vi "Data_get.vi"() -> ()   [LabVIEW 2009]
uses:
  <vilib>/Analysis/2dsp.llb/Real FFT.vi
  <vilib>/Analysis/NI_AALPro.lvlib
panel:
  in  "Auto":bool caption="Autosave"
  in  "FFT every#":u32=1 min=1 max=1000 step=1
  in  "#steps":u32=1 min=1 step=1
  in  "f step (MHz)":dbl=0.0003 min=0.00025 max=67.0 step=1e-06 format="%#.12f"
  in  "ps/point":T1(ring)
  in  "ns/div":T2(ring)
  out "Current sweep":u32=1 min=1 max=1000 step=1
  in  "Ext":string="ccd"
  out "f cur. (MHz)":string
  in  "Name":string="trace"
  in  "Folder":path
  in  "#Sweeps":u32=1 min=1 max=1000 step=1
  in  "Ampl. (dBm)":dbl min=-135.0 max=30.0 step=0.5 format="%#_8g"
  in  "f start (MHz)":dbl=0.0003 min=0.00025 max=67.0 step=1e-06 format="%#.12f"
  in  "Start":bool
  in  "Quit":bool
  in  "E8257D VISA Port":refnum<visa-resource-name>="GPIB0::1::INSTR"
  out "read time (ms)":u32
  out "#points":u32
  out "Busy":bool
  in  "Repetition rate (Hz)":ext=2.5
  in  "Chirp start (MHz)":ext=2.5
  in  "Filter up to (MHz)":ext=2.5
  in  "Amount of averagings":u32=10
  out "Data":dbl[](array[numeric])
  out "XY Graph 5":cluster{ext[], dbl[]}(graph)
  out "FFT (Im)":dbl[](array[numeric])
  out "FFT (Re)":dbl[](array[numeric])
  out "Final array":ext[][](array[numeric])
  out "size(s)":i32
  out "Oscilloscope Data":dbl[](array[numeric])
  in  "Channel Number":u16=1
  out "Oscilloscope graph":dbl[](graph)
  in  "Stop":bool
  in  "TDS VISA Port":refnum<visa-resource-name>="GPIB0::1::INSTR"
  # "TDS6000"
  # "E8257D"
  # "File Storage"
  # "Control"
  # "Spectrum data"
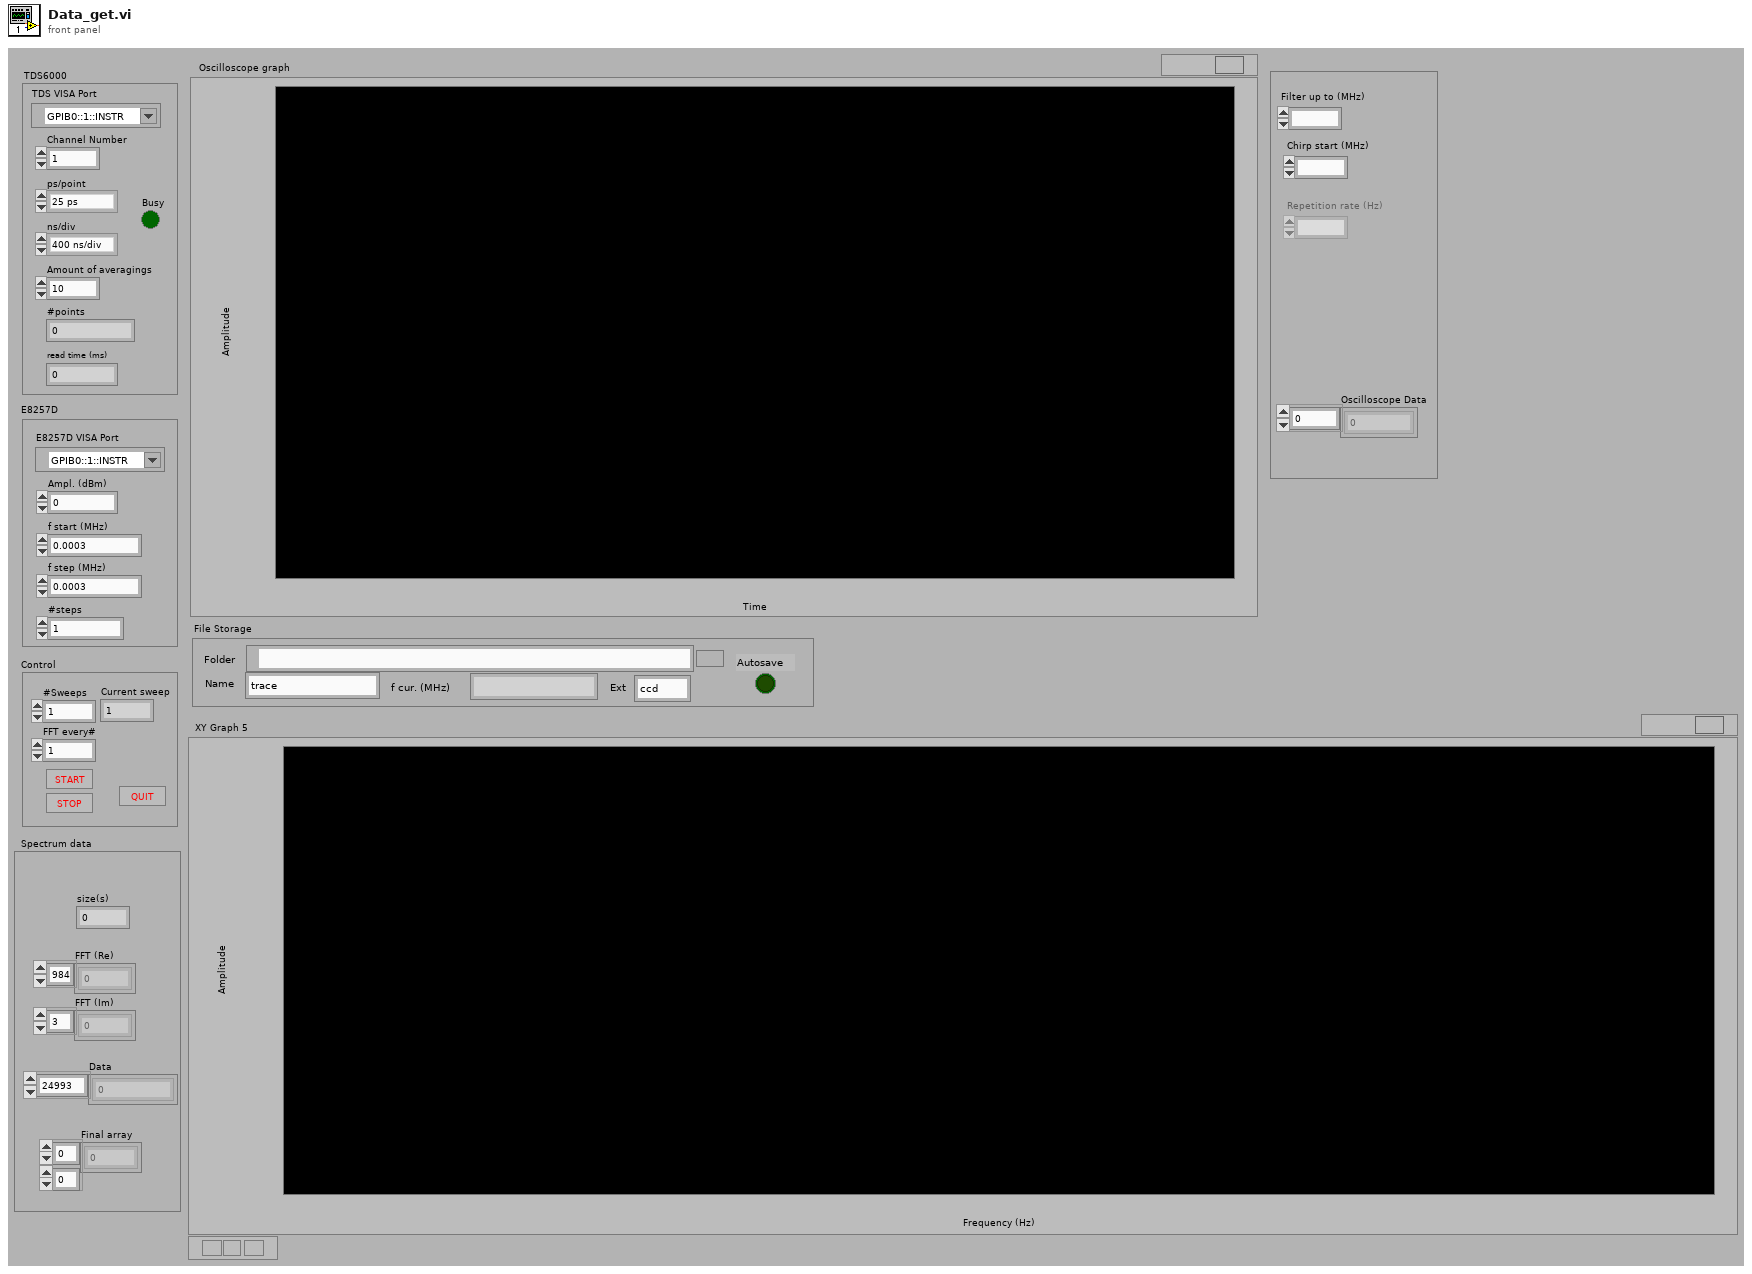
[diagram p1: front panel]
types:
  T1 = enum16{"25 ps", "50 ps", "100 ps", "200 ps", "400 ps", "800 ps", "2 ns"}
  T2 = enum16{"400 ns/div", "1 us/div", "2 us/div", "4 us/div", "10 us/div", "20 us/div"}
  T3 = enum16{"open", "replace", "create", "open or create", "replace or create", "replace or create with confirmation"}
  T4 = cluster{"Folder":path, "Name":string, "Ext":string}
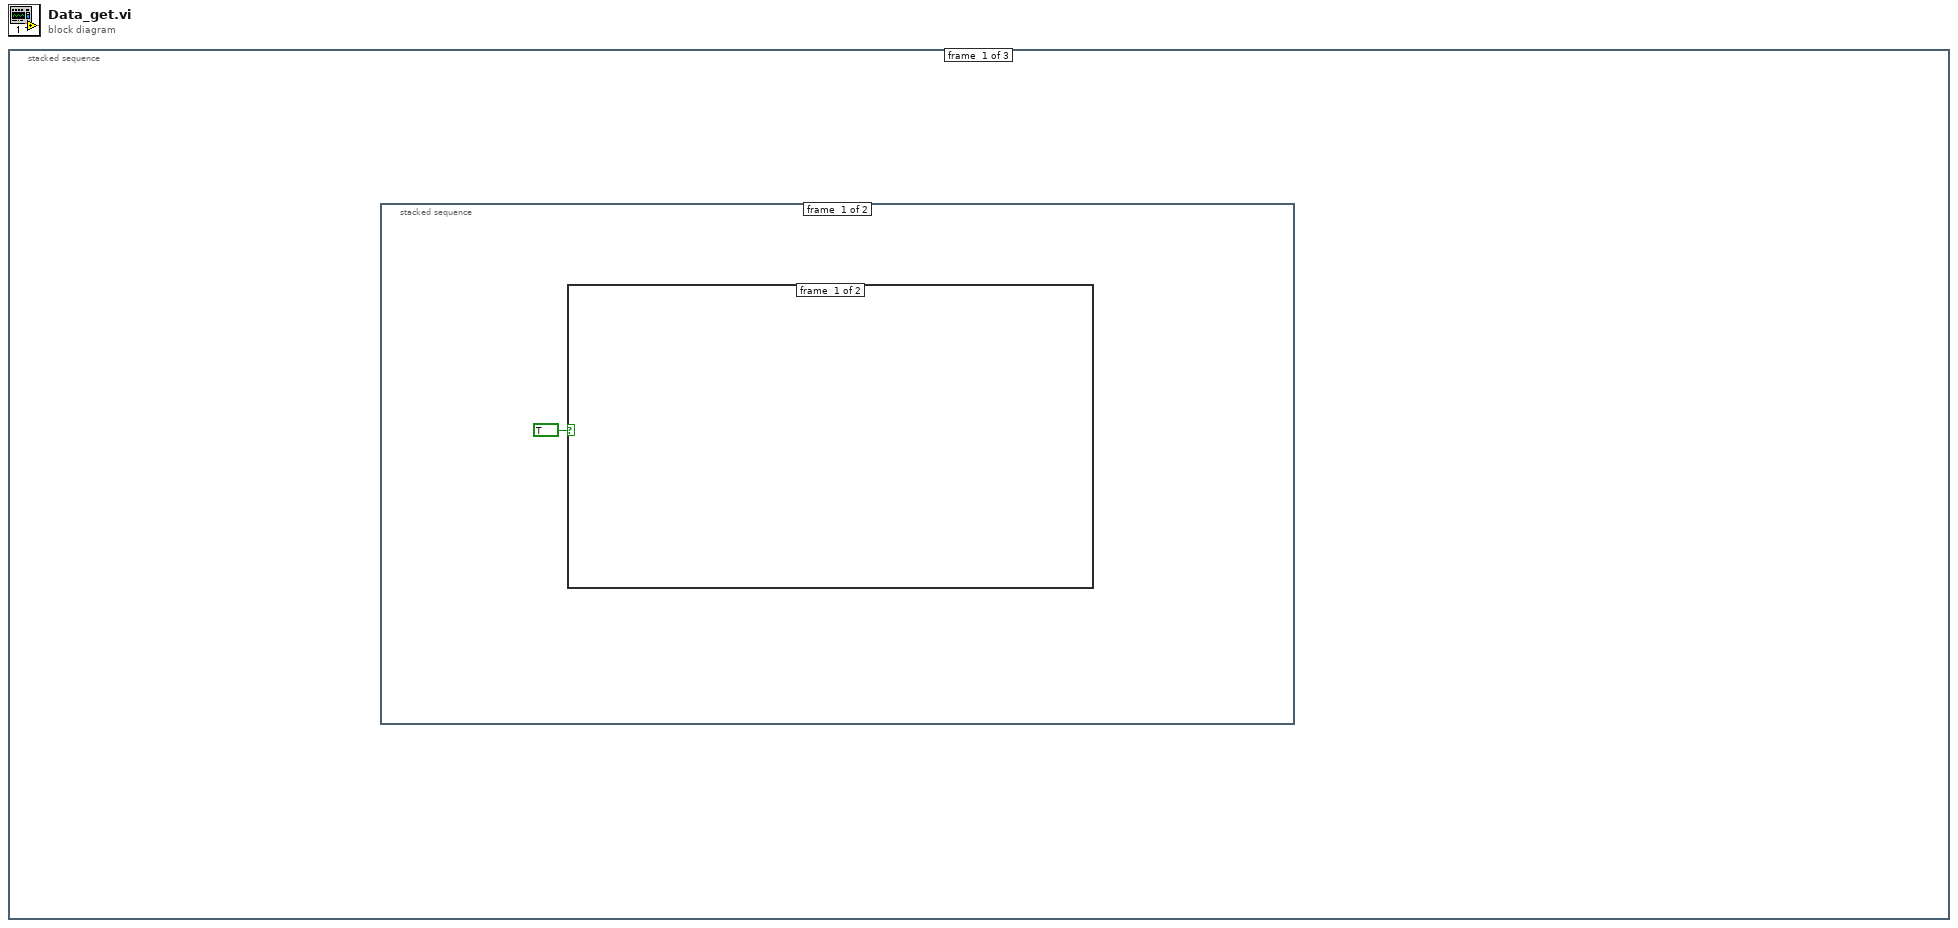
[diagram p0: block diagram]
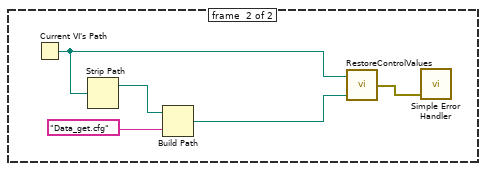
[diagram p2: hidden frame]
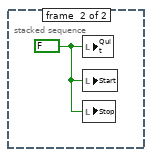
[diagram p3: hidden frame]
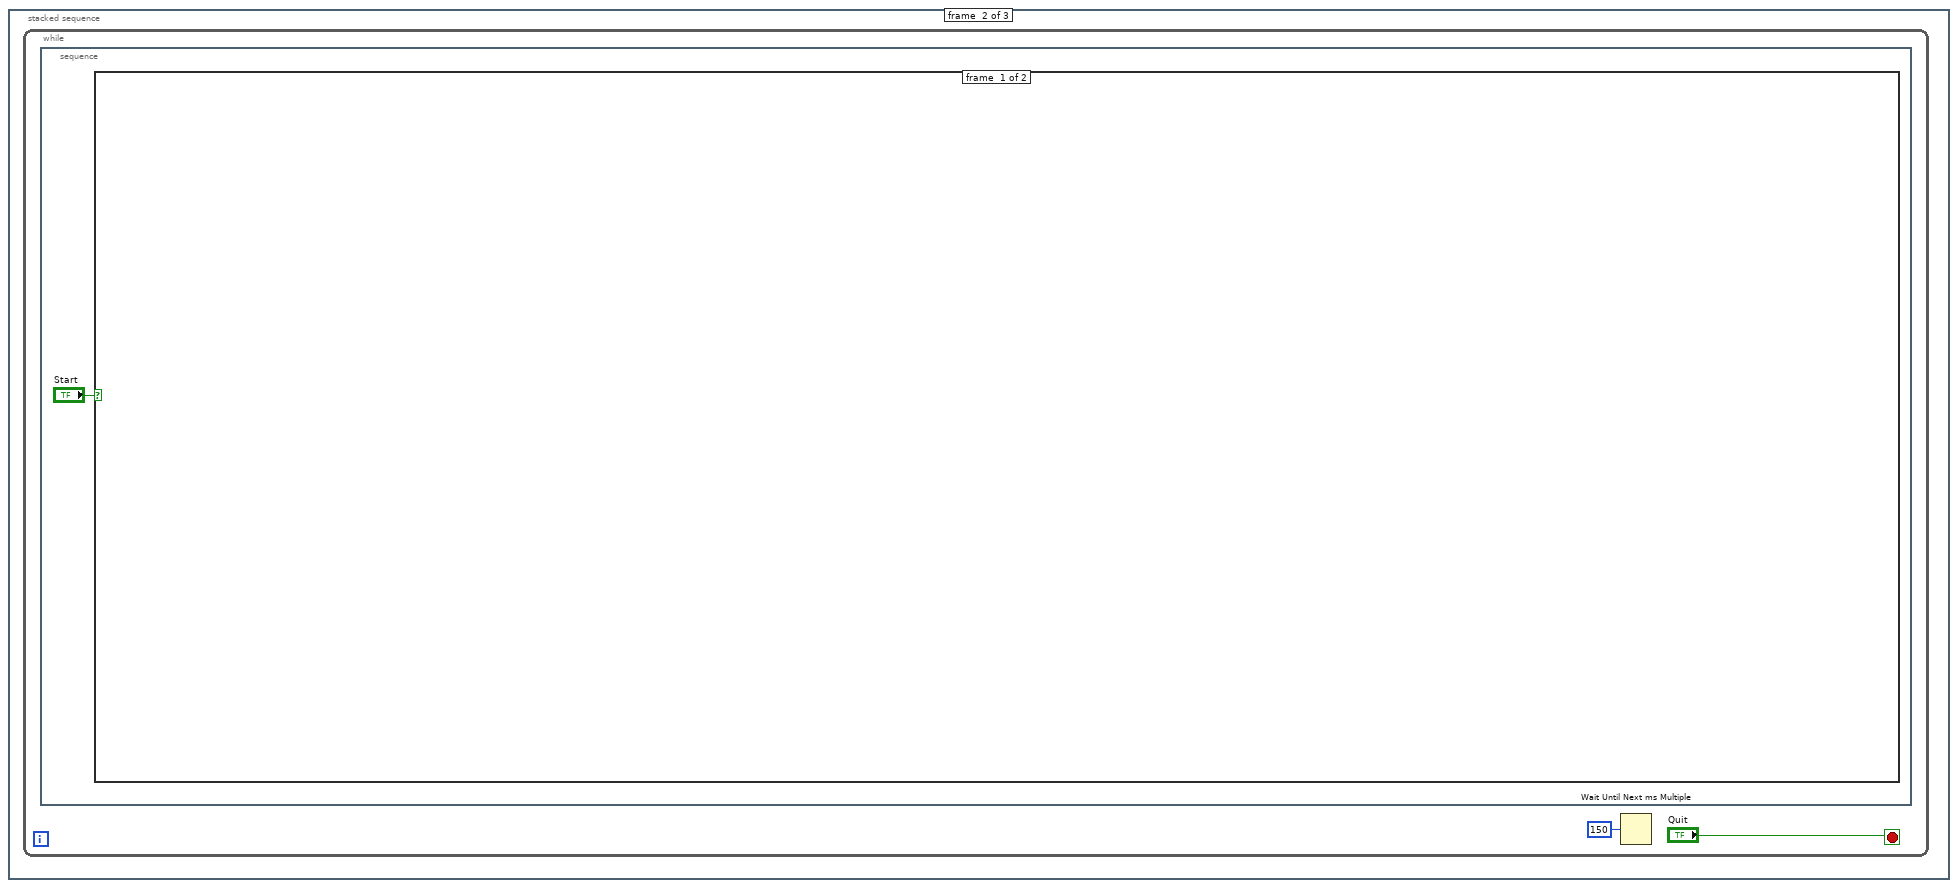
[diagram p4: hidden frame]
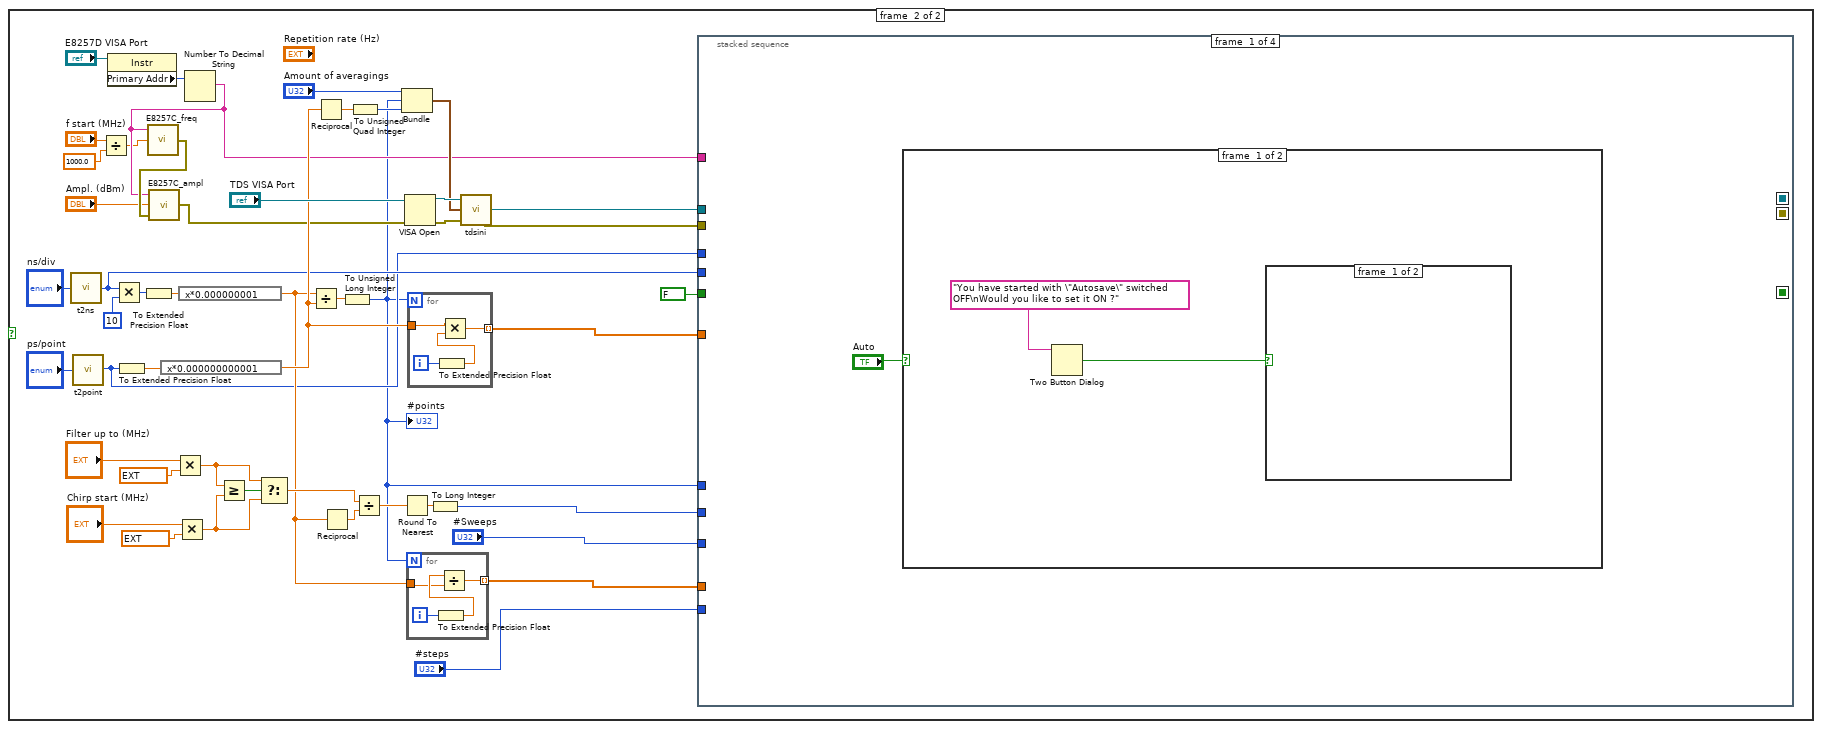
[diagram p5: hidden frame]
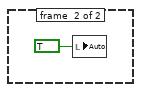
[diagram p6: hidden frame]
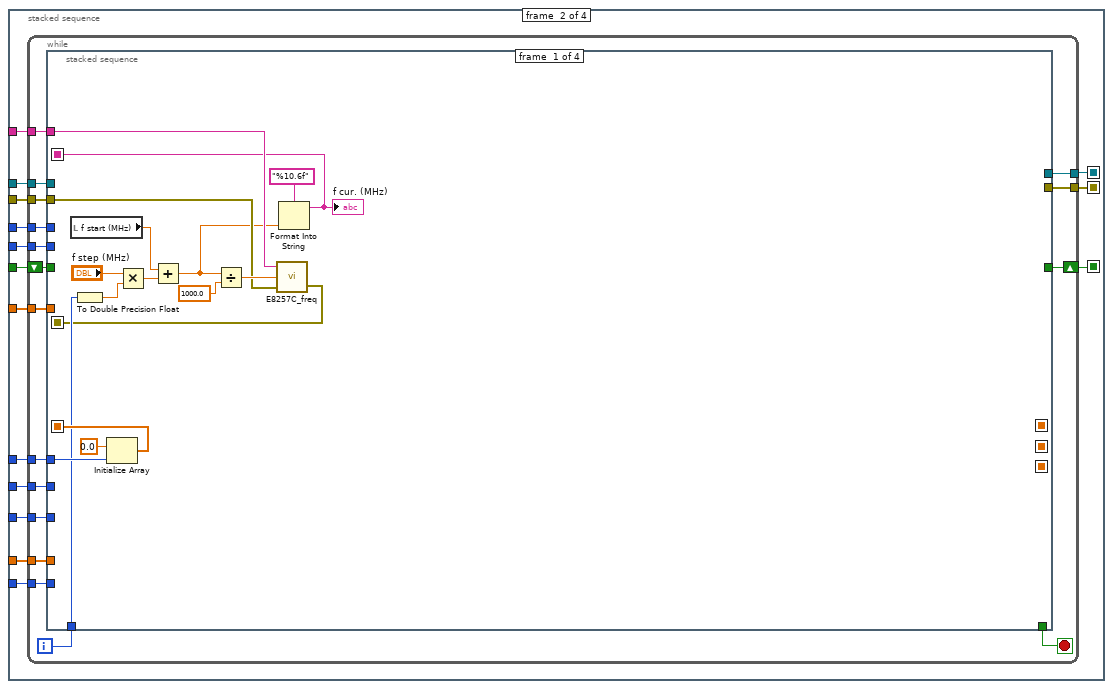
[diagram p8: hidden frame]
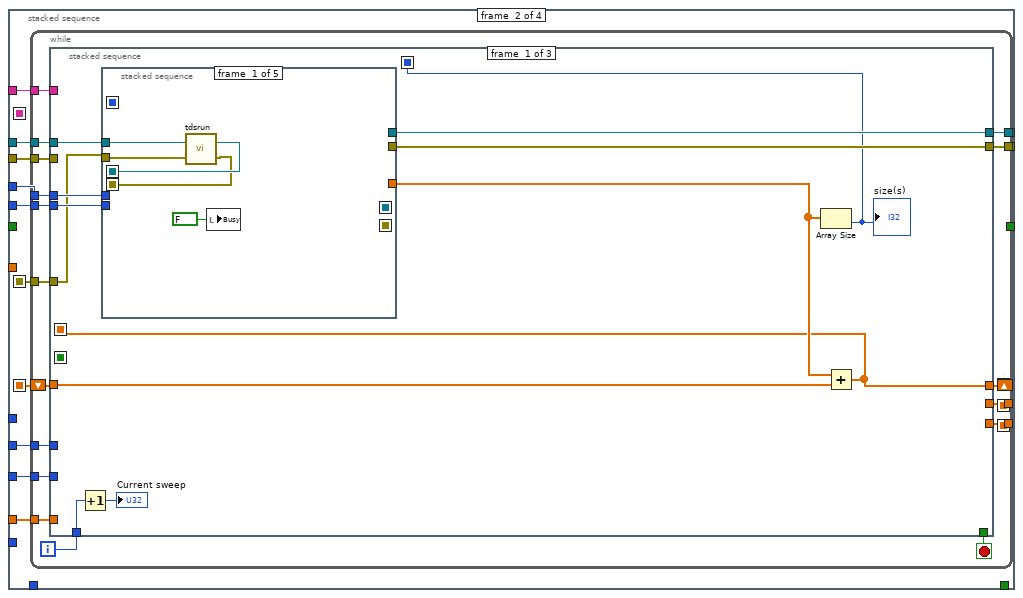
[diagram p9: hidden frame]
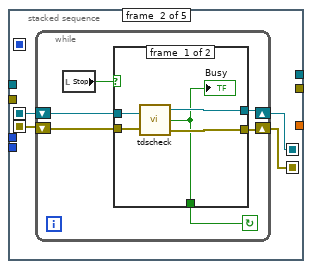
[diagram p10: hidden frame]
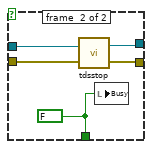
[diagram p11: hidden frame]
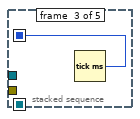
[diagram p12: hidden frame]
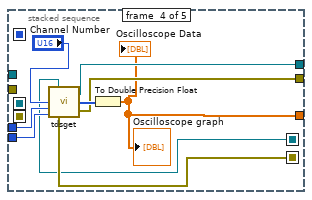
[diagram p13: hidden frame]
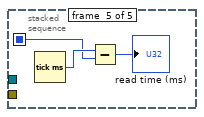
[diagram p14: hidden frame]
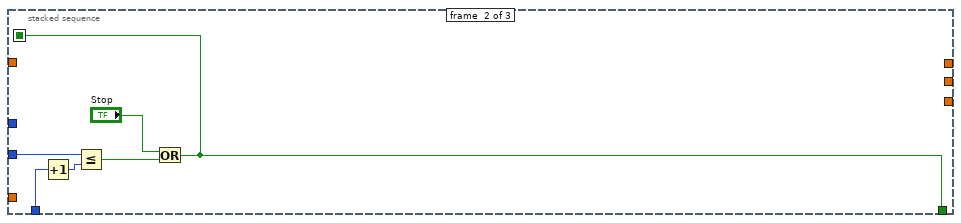
[diagram p15: hidden frame]
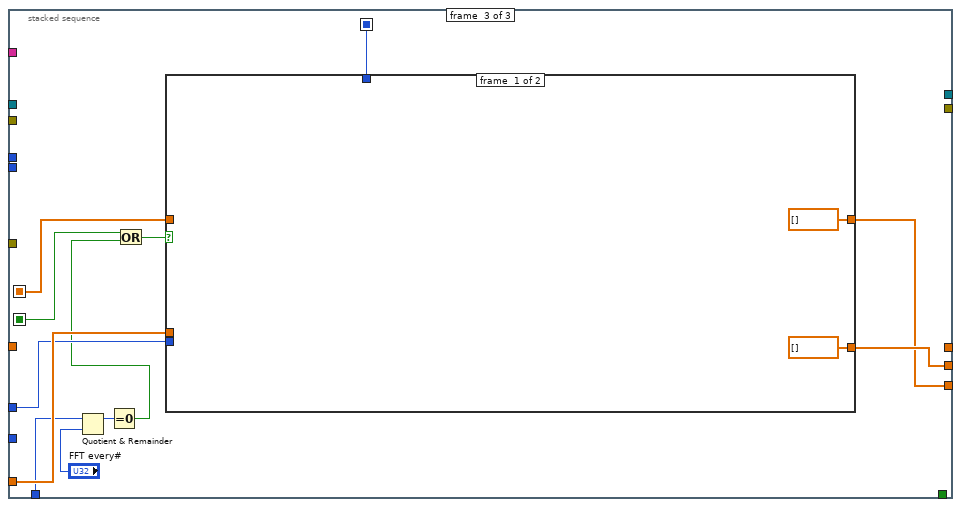
[diagram p16: hidden frame]
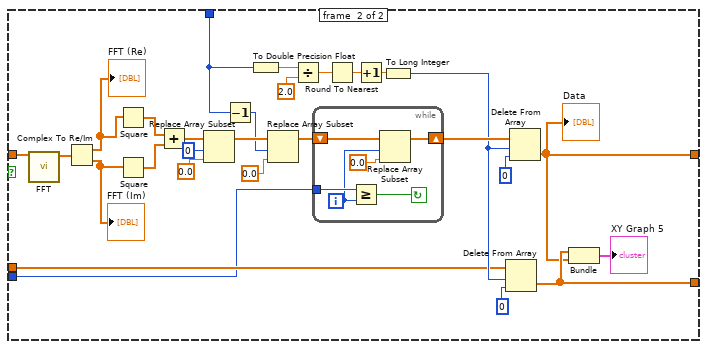
[diagram p17: hidden frame]
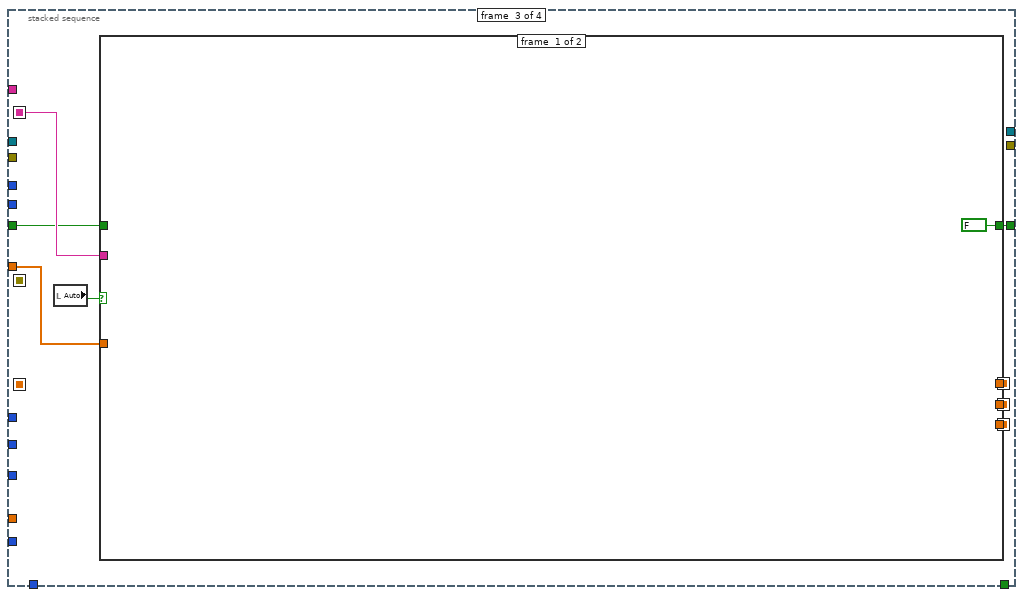
[diagram p18: hidden frame]
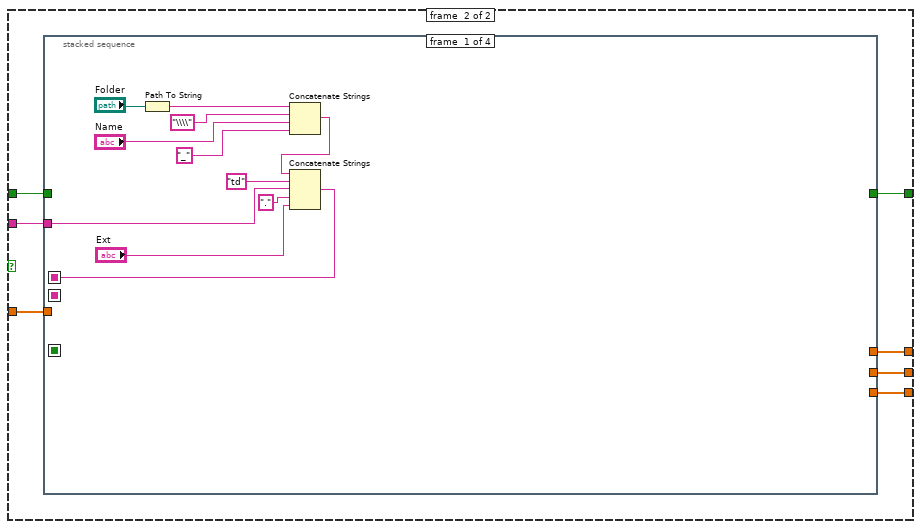
[diagram p19: hidden frame]
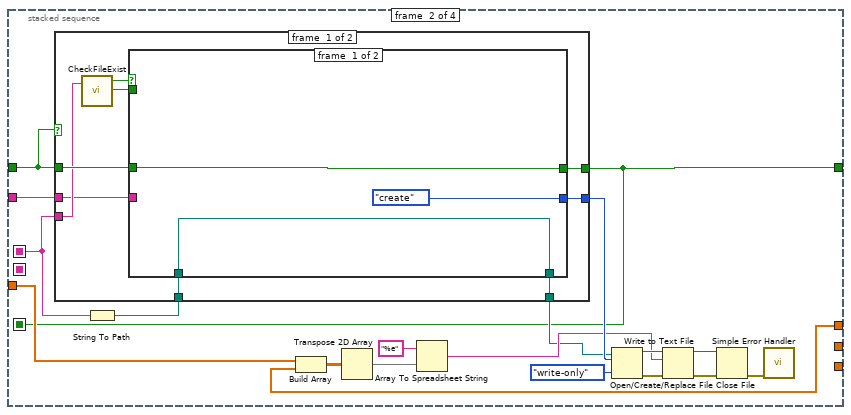
[diagram p20: hidden frame]
diagram:
  n1 = stacked-sequence {
    frame #0 {
      n2 = stacked-sequence {
        frame #0 {
          n3 = case shown="True" TRUE {
            frame #0 {
            }
            frame #1 {
              n4 = Current VI's Path() -> (path=w2:path)
              n5 = Strip Path(path=w2) -> (stripped path=w3:path)  [unwired: 1 out]
              n6 = Build Path(base path=w3, name or relative path="Data_get.cfg") -> (appended path=w5:path)
              n7 = call "RestoreControlValues.vi"("file path"=w5, "vi path"=w2) -> ("error out"=w4:errorcluster)
              n8 = call <vilib>:"Simple Error Handler.vi"("error in (no error)"=w4) -> ()  [unwired: 4 in, 5 out]
            }
          }
        }
        frame #1 {
          w7 = FALSE ("Quit")
          n9 = local write "Quit"(w7) -> ()
          n10 = local write "Start"(w7) -> ()
          n11 = local write "Stop"(w7) -> ()
        }
      }
    }
    frame #1 {
      n12 = while {
        stop <- "Quit" stop-if-true
        n13 = stacked-sequence {
          frame #0 {
            n14 = case shown="True" "Start" {
              frame #0 {
              }
              frame #1 {
                n15 = call "t2ns.vi"("t/div"="ns/div") -> ("ns/div"=w17:u32)
                n16 = call "t2point.vi"("t/point"="ps/point") -> ("ps/point"=w15:u32)
                n17 = Divide(x="f start (MHz)", y=1000.0) -> (x/y=w20:dbl)
                n18 = property class="Instr"(reference="E8257D VISA Port") -> ("Primary Addr"=w27:u16)  [unwired: 1 in, 2 out]
                n19 = Multiply(x=w17, y=u32 10) -> (x*y=w51:u32)
                n20 = To Extended Precision Float(1:w15) -> (0:w48:ext)
                n21 = To Extended Precision Float(1:w51) -> (0:w49:ext)
                n22 = expression code="x*0.000000000001"(w48) -> (w33:ext)
                n23 = Multiply(x="Filter up to (MHz)", y=ext 1000000.0) -> (x*y=w39:ext)
                n24 = Multiply(x="Chirp start (MHz)", y=ext 1000000.0) -> (x*y=w36:ext)
                n25 = expression code="x*0.000000001"(w49) -> (w29:ext)
                n26 = Number To Decimal String(number=w27) -> (decimal integer string=w24:string)  [unwired: 1 in]
                n27 = call "E8257C_freq.vi"("Frequency GHz"=w20, "GPIB address"=w24) -> ("error out"=w25:errorcluster)  [unwired: 1 in]
                n28 = call "E8257C_ampl.vi"("error in"=w25, "Amplitude dBm"="Ampl. (dBm)", "GPIB address"=w24) -> ("error out"=w23:errorcluster)
                n29 = Greater Or Equal?(x=w39, y=w36) -> (x >= y?=w47:bool)
                n30 = Select(t=w39, s=w47, f=w36) -> (s? t:f=w45:ext)
                n31 = Divide(x=w29, y=w33) -> (x/y=w50:ext)
                n32 = Reciprocal(x=w33) -> (1/x=w31:ext)
                n33 = Reciprocal(x=w29) -> (1/x=w46:ext)
                n34 = To Unsigned Long Integer(number=w50) -> (unsigned 32bit integer=w13:u32)
                "#points" <- w13
                n35 = To Unsigned Quad Integer(1:w31) -> (0:w32:u64)
                n36 = Divide(x=w45, y=w46) -> (x/y=w44:ext)
                n37 = Bundle("Amount of averagings"="Amount of averagings", w13, w32) -> (w34:cluster{"Amount of averagings ":u32, u32, u64})  [unwired: 1 in]
                n38 = Round To Nearest(number=w44) -> (nearest integer value=w43:ext)
                n39 = VISA Open(error in (no error)=w23, VISA resource name="TDS VISA Port") -> (VISA resource name=w54:refnum<visa-resource-name>, error out=w55:errorcluster)  [unwired: 3 in]
                n40 = for {
                  N: w13 -> [_]
                  tunnel: w29 -> [w420]
                  tunnel: [w422] -> w30 mode=indexing
                  i -> [w423]
                  n41 = To Extended Precision Float(1:w423) -> (0:w421:ext)
                  n42 = Divide(x=w421, y=w420) -> (x/y=w422:ext)
                }
                n43 = for {
                  N: w13 -> [_]
                  tunnel: w33 -> [w425]
                  tunnel: [w424] -> w18 mode=indexing
                  i -> [w427]
                  n44 = To Extended Precision Float(1:w427) -> (0:w426:ext)
                  n45 = Multiply(x=w425, y=w426) -> (x*y=w424:ext)
                }
                n46 = To Long Integer(number=w43) -> (32bit integer=w42:i32)
                n47 = call "tdsini.vi"("Error In (No Error)"=w55, "Acq_par"=w34, "VISA Port In"=w54) -> ("Error Out"=w56:errorcluster, "VISA Port Out"=w57:refnum<visa-resource-name>)
                n48 = stacked-sequence {
                  seq-local: [_ w68 _ _] -> [_ _ w381 _]
                  seq-local: [_ w67 _ _] -> [_ _ w380 _]
                  seq-local: [_ w62 _ _] -> [_ _ _ w382]
                  tunnel: w57 -> [_ w76 _ _]
                  tunnel: w56 -> [_ w75 _ _]
                  tunnel: w15 -> [_ w74 _ _]
                  tunnel: w17 -> [_ w73 _ _]
                  tunnel: w42 -> [_ w72 _ _]
                  tunnel: w30 -> [_ w71 _ _]
                  tunnel: w24 -> [_ w70 w378 _]
                  tunnel: "#Sweeps" -> [_ w69 _ _]
                  tunnel: w18 -> [_ w64 _ _]
                  tunnel: w13 -> [_ w66 _ _]
                  tunnel: "#steps" -> [_ w65 _ _]
                  tunnel: FALSE -> [_ w63 _ _]
                  frame #0 {
                    n49 = case shown="False" "Auto" {
                      frame #0 {
                        n50 = Two Button Dialog(message="You have started with \"Autosave\" switched OFF\nWould you like to set it ON ?") -> (T button?=w59:bool)  [unwired: 2 in]
                        n51 = case shown="True" w59 {
                          frame #0 {
                          }
                          frame #1 {
                            n52 = local write "Auto"(TRUE) -> ()
                          }
                        }
                      }
                      frame #1 {
                      }
                    }
                  }
                  frame #1 {
                    n53 = while {
                      tunnel: w76 -> [w93]
                      tunnel: w75 -> [w92]
                      tunnel: w74 -> [w91]
                      tunnel: w73 -> [w90]
                      tunnel: w72 -> [w89]
                      tunnel: w71 -> [w88]
                      tunnel: w70 -> [w87]
                      tunnel: w69 -> [w86]
                      tunnel: [w85] -> w68
                      tunnel: [w84] -> w67
                      tunnel: w66 -> [w83]
                      tunnel: w65 -> [w81]
                      tunnel: w64 -> [w79]
                      shift-right: [w77] -> w62
                      shift-left: w63 -> [w78]
                      i -> [w82]
                      stop <- w80 stop-if-true
                      n54 = stacked-sequence {
                        seq-local: [w108 _ _ _] -> [_ w114 _ _]
                        seq-local: [w97 _ _ _] -> [_ w113 _ _]
                        seq-local: [_ w112 _ _] -> [_ _ w252 _]
                        seq-local: [_ w111 _ _] -> [_ _ w251 _]
                        seq-local: [_ w110 _ _] -> [_ _ w250 _]
                        seq-local: [w94 _ _ _] -> [_ _ w249 _]
                        tunnel: w93 -> [_ w124 _ _]
                        tunnel: w92 -> [w98 w123 _ _]
                        tunnel: w91 -> [_ w122 _ _]
                        tunnel: w90 -> [_ w121 _ _]
                        tunnel: w89 -> [_ w120 _ _]
                        tunnel: w88 -> [_ w119 _ _]
                        tunnel: w87 -> [w99 w118 _ _]
                        tunnel: w86 -> [_ w117 _ _]
                        tunnel: [_ w116 _ _] -> w85
                        tunnel: [_ w115 _ _] -> w84
                        tunnel: w83 -> [w107 _ _ _]
                        tunnel: w82 -> [w102 _ _ w374]
                        tunnel: w81 -> [_ _ _ w373]
                        tunnel: [_ _ _ w372] -> w80
                        tunnel: w79 -> [_ _ w253 _]
                        tunnel: w78 -> [_ _ w247 _]
                        tunnel: [_ _ w246 _] -> w77
                        frame #0 {
                          n55 = local read "f start (MHz)"() -> (w100:dbl)
                          n56 = To Double Precision Float(number=w102) -> (double precision float=w103:dbl)
                          n57 = Initialize Array(0.0 ("element"), w107) -> (w108:dbl[])
                          n58 = Multiply(x="f step (MHz)", y=w103) -> (x*y=w101:dbl)
                          n59 = Add(x=w100, y=w101) -> (x+y=w96:dbl)
                          n60 = Divide(x=w96, y=1000.0) -> (x/y=w106:dbl)
                          n61 = call "E8257C_freq.vi"("error in"=w98, "Frequency GHz"=w106, "GPIB address"=w99) -> ("error out"=w97:errorcluster)
                          n62 = Format Into String(format string="%10.6f", w96) -> (resulting string=w94:string)  [unwired: 2 in, 1 out]
                          "f cur. (MHz)" <- w94
                        }
                        frame #1 {
                          n63 = while {
                            tunnel: [w138] -> w115
                            tunnel: [w139] -> w116
                            tunnel: w123 -> [w140]
                            tunnel: w124 -> [w141]
                            tunnel: w122 -> [w137]
                            tunnel: w121 -> [w136]
                            tunnel: w119 -> [w134]
                            tunnel: w120 -> [w135]
                            tunnel: w118 -> [w131]
                            tunnel: w117 -> [w130]
                            shift-right: [w128] -> w112
                            shift-left: w114 -> [w129]
                            tunnel: [w127] -> w111
                            tunnel: w113 -> [w126]
                            tunnel: [w125] -> w110
                            i -> [w133]
                            stop <- w132 stop-if-true
                            n64 = stacked-sequence {
                              seq-local: [w142 _ _] -> [_ _ w209]
                              seq-local: [w143 _ _] -> [_ _ w208]
                              seq-local: [_ w192 _] -> [_ _ w199]
                              tunnel: w141 -> [w153 _ _]
                              tunnel: w140 -> [_ _ _]
                              tunnel: [w152 _ _] -> w139
                              tunnel: [w151 _ _] -> w138
                              tunnel: w137 -> [w150 _ _]
                              tunnel: w136 -> [w149 _ _]
                              tunnel: w135 -> [_ _ w206]
                              tunnel: w134 -> [_ _ w207]
                              tunnel: w133 -> [w146 w197 w203]
                              tunnel: [_ w192 _] -> w132
                              tunnel: w131 -> [_ _ _]
                              tunnel: w130 -> [_ w194 _]
                              tunnel: w129 -> [w148 _ _]
                              tunnel: [w143 _ _] -> w128
                              tunnel: [_ _ w205] -> w127
                              tunnel: w126 -> [w145 _ _]
                              tunnel: [_ _ w204] -> w125
                              frame #0 {
                                n65 = Increment(x=w146) -> (x+1=→"Current sweep":i32)
                                n66 = stacked-sequence {
                                seq-local: [w156 _ _ _ _] -> [_ w162 _ _ _]
                                seq-local: [w155 _ _ _ _] -> [_ w161 _ _ _]
                                seq-local: [_ w159 _ _ _] -> [_ _ _ w181 _]
                                seq-local: [_ w160 _ _ _] -> [_ _ _ w180 _]
                                seq-local: [_ _ w179 _ _] -> [_ _ _ _ w190]
                                tunnel: w153 -> [w157 _ _ _ _]
                                tunnel: w145 -> [w158 _ _ _ _]
                                tunnel: [_ _ _ w187 _] -> w152
                                tunnel: [_ _ _ w186 _] -> w151
                                tunnel: w150 -> [_ _ _ w184 _]
                                tunnel: w149 -> [_ _ _ w183 _]
                                tunnel: [_ _ _ w182 _] -> w144
                                frame #0 {
                                n67 = call "tdsrun.vi"("Error In (No Error)"=w158, "VISA Port In"=w157) -> ("Error Out"=w155:errorcluster, "VISA Port Out"=w156:refnum<visa-resource-name>)
                                n68 = local write "Busy"(FALSE ("Busy")) -> ()
                                }
                                frame #1 {
                                n69 = while {
                                shift-right: [w166] -> w160
                                shift-left: w162 -> [w167]
                                shift-right: [w165] -> w159
                                shift-left: w161 -> [w168]
                                stop <- w164 continue-if-true
                                n70 = local read "Stop"() -> (w163:bool)
                                n71 = case shown="True" w163 {
                                tunnel: w168 -> [w173 w177]
                                tunnel: w167 -> [w172 w178]
                                tunnel: [w171 w175] -> w166
                                tunnel: [w170 w176] -> w165
                                tunnel: [w169 w174] -> w164
                                frame #0 {
                                n72 = call "tdscheck.vi"("VISA Port In"=w172, "Error In (No Error)"=w173) -> ("VISA Port Out"=w171:refnum<visa-resource-name>, "busy"=w169:bool, "Error Out"=w170:errorcluster)
                                "Busy" <- w169
                                }
                                frame #1 {
                                w174 = FALSE ("busy")
                                n73 = call "tdsstop.vi"("Error In (No Error)"=w177, "VISA Port In"=w178) -> ("Error Out"=w176:errorcluster, "VISA Port Out"=w175:refnum<visa-resource-name>)
                                n74 = local write "Busy"(w174) -> ()
                                }
                                }
                                }
                                }
                                frame #2 {
                                n75 = Tick Count (ms)() -> (millisecond timer value=w179:u32)
                                }
                                frame #3 {
                                n76 = call "tdsget.vi"("VISA Port In"=w180, "Channel Number"="Channel Number", "ps/point"=w184, "ns/div"=w183, "Error In (No Error)"=w181) -> ("VISA Port Out"=w187:refnum<visa-resource-name>, "TDS Data"=w188:u16[], "Error Out"=w186:errorcluster)  [unwired: 8 in]
                                n77 = To Double Precision Float(number=w188) -> (double precision float=w182:dbl[])
                                "Oscilloscope graph" <- w182
                                "Oscilloscope Data" <- w182
                                }
                                frame #4 {
                                n78 = Tick Count (ms)() -> (millisecond timer value=w191:u32)
                                n79 = Subtract(x=w191, y=w190) -> (x-y=→"read time (ms)":u32)
                                }
                                }
                                n80 = Array Size(array=w144) -> (size(s)=w142:i32)
                                "size(s)" <- w142
                                n81 = Add(x=w144, y=w148) -> (x+y=w143:dbl[])
                              }
                              frame #1 {
                                n82 = Increment(x=w197) -> (x+1=w193:i32)
                                n83 = Less Or Equal?(x=w194, y=w193) -> (x <= y?=w196:bool)
                                n84 = Or(x="Stop", y=w196) -> (x .or. y?=w192:bool)
                              }
                              frame #2 {
                                n85 = Quotient & Remainder(x=w203, y="FFT every#") -> (x-y*floor(x/y)=w201:u32)  [unwired: 1 out]
                                n86 = Equal To 0?(x=w201) -> (x = 0?=w198:bool)
                                n87 = Or(x=w199, y=w198) -> (x .or. y?=w200:bool)
                                n88 = case shown="True" w200 {
                                tunnel: w209 -> [_ w217]
                                tunnel: w208 -> [_ w216]
                                tunnel: w207 -> [_ w215]
                                tunnel: w206 -> [_ w214]
                                tunnel: [ext[] [] w213] -> w205
                                tunnel: [dbl[] [] w212] -> w204
                                frame #0 {
                                }
                                frame #1 {
                                n89 = call-poly <vilib>:"FFT.vi"("X"=w216) -> ("FFT {X}"=w239:cdb[])  [unwired: 9 in, 1 out]
                                n90 = Complex To Re/Im(x + iy=w239) -> (x=w238:dbl[], y=w237:dbl[])
                                "FFT (Re)" <- w238
                                "FFT (Im)" <- w237
                                n91 = Square(x=w238) -> (x^2=w236:dbl[])
                                n92 = Square(x=w237) -> (x^2=w235:dbl[])
                                n93 = Add(x=w236, y=w235) -> (x+y=w231:dbl[])
                                n94 = Replace Array Subset(array=w231, new element=0.0 ("new element/subarray"), index=0) -> (w230:dbl[])
                                n95 = Decrement(x=w217) -> (x-1=w229:i32)
                                n96 = To Double Precision Float(number=w217) -> (double precision float=w225:dbl)
                                n97 = Replace Array Subset(array=w230, new element=0.0 ("new element/subarray"), index=w229) -> (w227:dbl[])
                                n98 = Divide(x=w225, y=2.0) -> (x/y=w223:dbl)
                                n99 = while {
                                tunnel: w214 -> [w244]
                                shift-right: [w242] -> w226
                                shift-left: w227 -> [w243]
                                i -> [w241]
                                stop <- w245 continue-if-true
                                n100 = Greater Or Equal?(x=w244, y=w241) -> (x >= y?=w245:bool)
                                n101 = Replace Array Subset(array=w243, new element=0.0 ("new element/subarray"), index=w241) -> (w242:dbl[])
                                }
                                n102 = Round To Nearest(number=w223) -> (nearest integer value=w222:dbl)
                                n103 = Increment(x=w222) -> (x+1=w221:dbl)
                                n104 = To Long Integer(number=w221) -> (32bit integer=w218:i32)
                                n105 = Delete From Array(array=w215, length=w218, index=0) -> (deleted portion=w213:ext[])  [unwired: 1 out]
                                n106 = Delete From Array(array=w226, length=w218, index=0) -> (deleted portion=w212:dbl[])  [unwired: 1 out]
                                "Data" <- w212
                                n107 = Bundle(w213, w212) -> (→"XY Graph 5":cluster{ext[], dbl[]})  [unwired: 1 in]
                                }
                                }
                              }
                            }
                          }
                        }
                        frame #2 {
                          n108 = local read "Auto"() -> (w248:bool)
                          n109 = case shown="True" w248 {
                            tunnel: w253 -> [_ w261]
                            tunnel: w252 -> [_ w260]
                            tunnel: w251 -> [_ w259]
                            tunnel: w250 -> [_ w258]
                            tunnel: w249 -> [_ w257]
                            tunnel: w247 -> [_ w256]
                            tunnel: [FALSE w255] -> w246
                            frame #0 {
                            }
                            frame #1 {
                              n110 = stacked-sequence {
                                seq-local: [w262 _ _ _] -> [_ w287 _ _]
                                seq-local: [_ _ w342 _] -> [_ _ _ w363]
                                seq-local: [_ w274 _ _] -> [_ _ _ w354]
                                tunnel: w261 -> [_ w289 _ _]
                                tunnel: w260 -> [_ w276 _ _]
                                tunnel: w259 -> [_ _ _ w366]
                                tunnel: w258 -> [_ _ _ w365]
                                tunnel: w257 -> [w264 w275 w344 _]
                                tunnel: w256 -> [_ w279 _ _]
                                tunnel: [_ w274 _ _] -> w255
                                frame #0 {
                                n111 = Path To String(path="Folder") -> (string=w272:string)
                                n112 = Concatenate Strings(w272, "\\\\" ("string"), "Name", "_") -> (w263:string)
                                n113 = Concatenate Strings(w263, "td", w264, ".", "Ext") -> (w262:string)
                                }
                                frame #1 {
                                n114 = String To Path(string=w287) -> (path=w278:path)
                                n115 = case shown="False" w279 {
                                tunnel: w287 -> [w293 _]
                                tunnel: [w298 w340] -> w274
                                tunnel: [w296 T3."replace or create" ("operation (0:open)")] -> w281
                                tunnel: w279 -> [w297 w340]
                                tunnel: w278 -> [w295 w339]
                                tunnel: [w294 w339] -> w277
                                tunnel: w275 -> [w292 _]
                                frame #0 {
                                n116 = call "CheckFileExist.vi"("Path"=w293) -> ("Exist"=w300:bool, "Overwrite"=w299:bool)  [unwired: 1 in, 1 out]
                                n117 = case shown="True" w300 {
                                tunnel: w299 -> [_ w309]
                                tunnel: [w303 w307] -> w298
                                tunnel: w297 -> [w303 _]
                                tunnel: [T3."create" ("operation (0:open)") w308] -> w296
                                tunnel: w295 -> [w301 w306]
                                tunnel: [w301 w305] -> w294
                                tunnel: w292 -> [_ w304]
                                frame #0 {
                                }
                                frame #1 {
                                n118 = case shown="True" w309 {
                                tunnel: [w312 T3."replace or create" ("operation (0:open)")] -> w308
                                tunnel: [w313 TRUE] -> w307
                                tunnel: w306 -> [_ w336]
                                tunnel: [w310 w336] -> w305
                                tunnel: w304 -> [w311 _]
                                frame #0 {
                                n119 = stacked-sequence {
                                tunnel: [_ _ FALSE] -> w313
                                tunnel: [_ _ T3."create" ("operation (0:open)")] -> w312
                                tunnel: w311 -> [_ w325 _]
                                tunnel: [_ w322 _] -> w310
                                frame #0 {
                                n120 = local read "Folder"() -> (w321:path)
                                n121 = local read "Name"() -> (w320:string)
                                n122 = local read "Ext"() -> (w319:string)
                                n123 = Bundle("Folder"=w321, "Name"=w320, "Ext"=w319) -> (w318:T4)  [unwired: 1 in]
                                n124 = call "ChangeFileName.vi"("input par"=w318) -> ("output par"=w317:T4)  [unwired: 1 out]
                                n125 = Unbundle(w317) -> ("Folder"=w316:path, "Name"=w315:string, "Ext"=w314:string)
                                n126 = local write "Folder"(w316) -> ()
                                n127 = local write "Name"(w315) -> ()
                                n128 = local write "Ext"(w314) -> ()
                                }
                                frame #1 {
                                n129 = local read "Folder"() -> (w330:path)
                                n130 = local read "Name"() -> (w329:string)
                                n131 = local read "Ext"() -> (w324:string)
                                n132 = Path To String(path=w330) -> (string=w333:string)
                                n133 = Concatenate Strings(w333, "\\\\" ("string"), w329, "_") -> (w326:string)
                                n134 = Concatenate Strings(w326, "td", w325, ".", w324) -> (w323:string)
                                n135 = String To Path(string=w323) -> (path=w322:path)
                                }
                                frame #2 {
                                }
                                }
                                }
                                frame #1 {
                                }
                                }
                                }
                                }
                                }
                                frame #1 {
                                }
                                }
                                n136 = Build Array(w289, w276) -> (w291:ext[][])
                                n137 = Transpose 2D Array(2D array=w291) -> (transposed array=w288:ext[][])
                                n138 = Array To Spreadsheet String(array=w288, 3:"%e") -> (spreadsheet string=w280:string)  [unwired: 1 in]
                                n139 = Open/Create/Replace File(file path (use dialog)=w277, operation (0:open)=w281, access (0:read/write)=enum16{"read/write", "read-only", "write-only"}."write-only") -> (refnum out=w283:refnum<file>, error out=w286:errorcluster)  [unwired: 3 in, 1 out]
                                n140 = Write to Text File(file (use dialog)=w283, text=w280, error in=w286) -> (refnum out=w284:refnum<file>, error out=w285:errorcluster)  [unwired: 1 in, 1 out]
                                n141 = Close File(refnum=w284, error in=w285) -> (error out=w273:errorcluster)  [unwired: 1 out]
                                n142 = call <vilib>:"Simple Error Handler.vi"("error in (no error)"=w273) -> ()  [unwired: 4 in, 5 out]
                                }
                                frame #2 {
                                n143 = local read "Folder"() -> (w346:path)
                                n144 = local read "Name"() -> (w345:string)
                                n145 = local read "Ext"() -> (w343:string)
                                n146 = Path To String(path=w346) -> (string=w352:string)
                                n147 = Concatenate Strings(w352, "\\\\" ("string"), w345, "_") -> (w347:string)
                                n148 = Concatenate Strings(w347, "sd", w344, ".", w343) -> (w342:string)
                                }
                                frame #3 {
                                n149 = To Extended Precision Float(1:w365) -> (0:w367:ext[])
                                n150 = String To Path(string=w363) -> (path=w356:path)
                                n151 = case shown="True" w354 {
                                tunnel: [T3."replace or create with confirmation" ("operation (0:open)") T3."replace or create" ("operation (0:open)")] -> w355
                                frame #0 {
                                }
                                frame #1 {
                                }
                                }
                                n152 = Build Array(w366, w367) -> (w364:ext[][])
                                n153 = Transpose 2D Array(2D array=w364) -> (transposed array=w368:ext[][])
                                "Final array" <- w368
                                n154 = Array To Spreadsheet String(array=w368, 3:"%e") -> (spreadsheet string=w357:string)  [unwired: 1 in]
                                n155 = Open/Create/Replace File(file path (use dialog)=w356, operation (0:open)=w355, access (0:read/write)=enum16{"read/write", "read-only", "write-only"}."write-only") -> (refnum out=w359:refnum<file>, error out=w362:errorcluster)  [unwired: 3 in, 1 out]
                                n156 = Write to Text File(file (use dialog)=w359, text=w357, error in=w362) -> (refnum out=w360:refnum<file>, error out=w361:errorcluster)  [unwired: 1 in, 1 out]
                                n157 = Close File(refnum=w360, error in=w361) -> (error out=w353:errorcluster)  [unwired: 1 out]
                                n158 = call <vilib>:"Simple Error Handler.vi"("error in (no error)"=w353) -> ()  [unwired: 4 in, 5 out]
                                }
                              }
                            }
                          }
                        }
                        frame #3 {
                          n159 = Increment(x=w374) -> (x+1=w376:i32)
                          n160 = Less Or Equal?(x=w373, y=w376) -> (x <= y?=w377:bool)
                          n161 = local read "Stop"() -> (w375:bool)
                          n162 = Or(x=w375, y=w377) -> (x .or. y?=w372:bool)
                        }
                      }
                    }
                  }
                  frame #2 {
                    n163 = call "E8257C_local.vi"("GPIB address"=w378) -> ("error out"=w379:errorcluster)  [unwired: 1 in]
                    n164 = call <vilib>:"Simple Error Handler.vi"("error in (no error)"=w379) -> ()  [unwired: 4 in, 5 out]
                    n165 = VISA Close(VISA resource name=w381, error in (no error)=w380) -> ()  [unwired: 1 out]
                  }
                  frame #3 {
                    n166 = local read "Auto"() -> (w383:bool)
                    n167 = case shown="True" w383 {
                      tunnel: w382 -> [_ w386]
                      frame #0 {
                      }
                      frame #1 {
                        n168 = local read "Channel Number"() -> (w416:u16)
                        n169 = local read "ps/point"() -> (w415:T1)
                        n170 = local read "ns/div"() -> (w414:T2)
                        n171 = local read "Amount of averagings"() -> (w413:u32)
                        n172 = local read "#Sweeps"() -> (w412:u32)
                        n173 = local read "Filter up to (MHz)"() -> (w411:ext)
                        n174 = local read "Chirp start (MHz)"() -> (w410:ext)
                        n175 = local read "Ampl. (dBm)"() -> (w409:dbl)
                        n176 = local read "f start (MHz)"() -> (w406:dbl)
                        n177 = local read "f step (MHz)"() -> (w405:dbl)
                        n178 = local read "#steps"() -> (w404:u32)
                        n179 = call "t2point.vi"("t/point"=w415) -> ("ps/point"=w407:u32)
                        n180 = call "t2ns.vi"("t/div"=w414) -> ("ns/div"=w408:u32)
                        n181 = local read "Folder"() -> (w400:path)
                        n182 = local read "Name"() -> (w399:string)
                        n183 = local read "Ext"() -> (w396:string)
                        n184 = Path To String(path=w400) -> (string=w403:string)
                        n185 = Format Into String(format string="Channel: %d\\nps/point: %d\\nns/div: %d\\nAmount of averagings: %d\\n#Sweeps: %d\\nFilter up to (MHz): %f\\nChirp start (MHz): %f\\nAmpl. (dBm): %f\\nf start (MHz): %f\\nf step (MHz): %f\\n#steps: %d\\n", w416, w407, w408, w413, w412, w411, w410, w409, w406, w405, w404) -> (resulting string=w387:string)  [unwired: 2 in, 1 out]
                        n186 = Concatenate Strings(w403, "\\\\" ("string"), w399, "_", "par", ".", w396) -> (w395:string)
                        n187 = case shown="False" w386 {
                          tunnel: [T3."replace or create with confirmation" ("operation (0:open)") T3."replace or create" ("operation (0:open)")] -> w385
                          frame #0 {
                          }
                          frame #1 {
                          }
                        }
                        n188 = String To Path(string=w395) -> (path=w389:path)
                        n189 = Open/Create/Replace File(file path (use dialog)=w389, operation (0:open)=w385, access (0:read/write)=enum16{"read/write", "read-only", "write-only"}."write-only") -> (refnum out=w391:refnum<file>, error out=w394:errorcluster)  [unwired: 3 in, 1 out]
                        n190 = Write to Text File(file (use dialog)=w391, text=w387, error in=w394) -> (refnum out=w392:refnum<file>, error out=w393:errorcluster)  [unwired: 1 in, 1 out]
                        n191 = Close File(refnum=w392, error in=w393) -> (error out=w390:errorcluster)  [unwired: 1 out]
                        n192 = call <vilib>:"Simple Error Handler.vi"("error in (no error)"=w390) -> ()  [unwired: 4 in, 5 out]
                      }
                    }
                    n193 = local write "Stop"(FALSE ("Stop")) -> ()
                  }
                }
              }
            }
          }
        }
        n194 = Wait Until Next ms Multiple(millisecond multiple=u32 150) -> ()  [unwired: 1 out]
      }
    }
    frame #2 {
      n195 = Current VI's Path() -> (path=w428:path)
      n196 = Strip Path(path=w428) -> (stripped path=w429:path)  [unwired: 1 out]
      n197 = Build Path(base path=w429, name or relative path="Data_get.cfg") -> (appended path=w431:path)
      n198 = call "SaveControlValues.vi"("file path"=w431, "vi path"=w428) -> ("error out"=w430:errorcluster)
      n199 = call <vilib>:"Simple Error Handler.vi"("error in (no error)"=w430) -> ()  [unwired: 4 in, 5 out]
    }
  }
